vi "Run Type Panel.vi"(7 "Sub Panel":refnum<vi>, 8 "error in (no error)":errorcluster, 11 "ColumnPanel in":refnum<class "ColumnPanel.lvclass">) -> (0 "error out":errorcluster, 3 "ColumnPanel out":refnum<class "ColumnPanel.lvclass">)   [LabVIEW 2020, in "Conditum-Tools.lvlib" / "ColumnPanel.lvclass"]
uses:
  ColumnPanel.lvclass
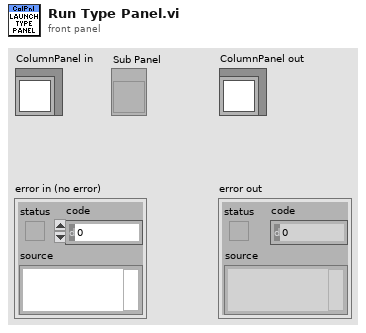
[diagram p1: front panel]
types:
  T1 = enum32{"invalid scope", "public", "private", "protected", "community"}
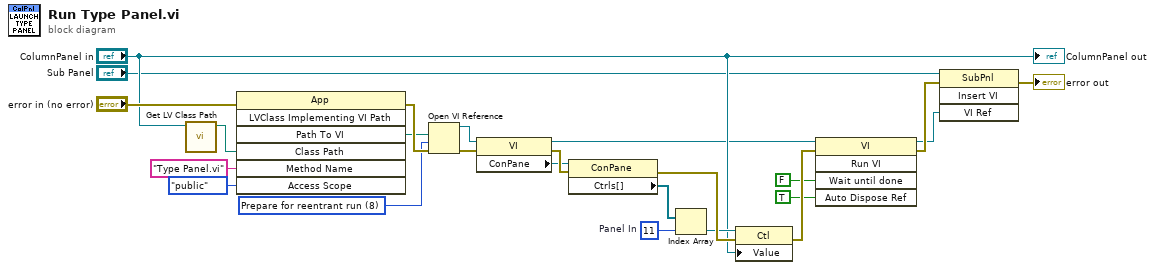
[diagram p0: block diagram]
diagram:
  w10 = 11  # Panel In
  w15 = 8 items=["Record modifications"=1, "Open templates for editing"=2, "Prompt user to save"=4, "Prepare for reentrant run"=8, "Prompt to find missing subVIs"=16, "Hide loading dialog box"=32, "Enable simultaneous calls"=64, "Prepare to call and forget"=128, "Simultaneous call and forget"=192, "Prepare to call and collect"=256, "Simultaneous call and collect"=320]
  n1 = call <vilib>:"Get LV Class Path.vi"("object"="ColumnPanel in") -> ("class path"=w19:path)  [unwired: 9 in, 1 out]
  n2 = invoke class="App" method="LVClass Implementing VI Path"(error in="error in (no error)", "Class Path"=w19, "Method Name"="Type Panel.vi", "Access Scope"=T1."public") -> (error out=w20:errorcluster, "Path To VI"=w16:path)  [unwired: 3 in, 5 out]
  n3 = Open VI Reference(vi path=w16, options=w15, error in (no error)=w20) -> (vi reference=w13:refnum<vi>, error out=w14:errorcluster)  [unwired: 3 in]
  n4 = property class="VI"(reference=w13, error in=w14) -> (reference out=w7:refnum<vi>, error out=w21:errorcluster, "ConPane"=w12:refnum<vi>)
  n5 = property class="ConPane"(reference=w12, error in=w21) -> (error out=w24:errorcluster, "Ctrls[]"=w11:refnum<vi>[])  [unwired: 1 out]
  n6 = Index Array(array=w11, index=w10) -> (element=w9:refnum<vi>)
  n7 = property class="Ctl"(reference=w9, error in=w24, "Value"="ColumnPanel in") -> (error out=w6:errorcluster)  [unwired: 1 out]
  n8 = invoke class="VI" method="Run VI"(reference=w7, error in=w6, "Wait until done"=FALSE ("Wait Until Done"), "Auto Dispose Ref"=TRUE ("Auto Dispose Reference")) -> (reference out=w2:refnum<vi>, error out=w23:errorcluster)  [unwired: 1 in, 3 out]
  n9 = invoke class="SubPnl" method="Insert VI"(reference="Sub Panel", error in=w23, "VI Ref"=w2) -> (error out=→"error out":errorcluster)  [unwired: 1 in, 3 out]
  "ColumnPanel out" <- "ColumnPanel in"
